vi "IRDistance w LED.vi"() -> ()   [LabVIEW 2017]
panel:
  in  "stop":bool
  out "interpolation value":dbl format="%0.2f"
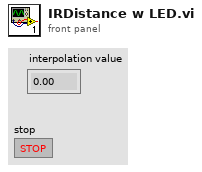
[diagram p1: front panel]
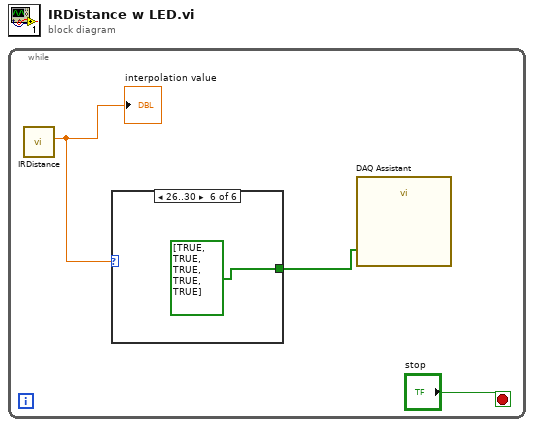
[diagram p0: block diagram]
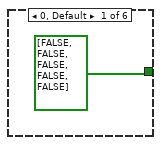
[diagram p2: hidden frame]
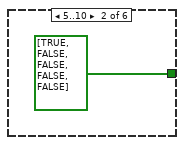
[diagram p3: hidden frame]
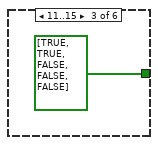
[diagram p4: hidden frame]
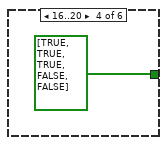
[diagram p5: hidden frame]
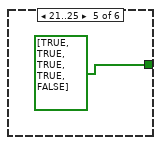
[diagram p6: hidden frame]
diagram:
  n1 = while {
    stop <- "stop" stop-if-true
    n2 = call "IRDistance.vi"() -> ("interpolation value"=w3:dbl)  [unwired: 11 in]
    "interpolation value" <- w3
    n3 = case shown="26..30" w3 {
      tunnel: [bool[] [FALSE, FALSE, FALSE, FALSE, FALSE] bool[] [TRUE, FALSE, FALSE, FALSE, FALSE] bool[] [TRUE, TRUE, FALSE, FALSE, FALSE] bool[] [TRUE, TRUE, TRUE, FALSE, FALSE] bool[] [TRUE, TRUE, TRUE, TRUE, FALSE] bool[] [TRUE, TRUE, TRUE, TRUE, TRUE]] -> w1
      frame 0, Default {
      }
      frame 5..10 {
      }
      frame 11..15 {
      }
      frame 16..20 {
      }
      frame 21..25 {
      }
      frame 26..30 {
      }
    }
    n4 = call "DAQ Assistant"("data"=w1) -> ()  [unwired: 17 in, 2 out]
  }
